vi "Get Annotation Style.vi"(0 "TTLControl in":refnum<class "TTLController.lvclass">, 11 "error in (no error)":errorcluster) -> (4 "TTLControl out":refnum<class "TTLController.lvclass">, 6 "Name":string, 8 "Style":T1, 10 "Active":bool, 15 "error out":errorcluster)   [LabVIEW 2015, in "TTLController.lvclass"]
uses:
  TTLController.lvclass
  FSM Graph VIs/LV Source/Classes/FSM.Annotation/Annotation Style.ctl
  TTLController.lvclass/TTLController.ctl
  FSM Graph VIs/LV Source/Classes/FSM.Annotation/FSM.Annotation.lvclass
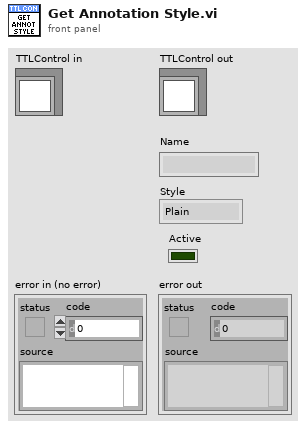
[diagram p1: front panel]
types:
  T1 = typedef "FSM.Annotation.lvclass/Annotation Style.ctl" = enum16{"Plain", "On", "Off", "On-Off"}
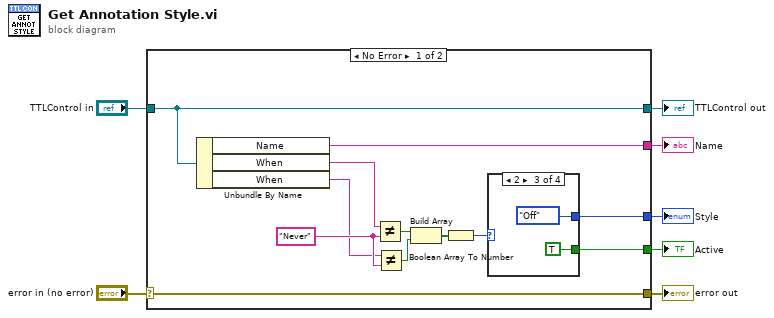
[diagram p0: block diagram]
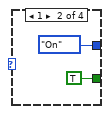
[diagram p3: hidden frame]
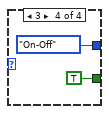
[diagram p4: hidden frame]
diagram:
  n1 = case shown="No Error" "error in (no error)" {
    selector: "error in (no error)" -> [w19 w27]
    tunnel: [w19 w27] -> w6
    tunnel: [w18 w26] -> w4
    tunnel: "TTLControl in" -> [w18 w26]
    tunnel: [w17 _] -> w3
    tunnel: [w9 _] -> w2
    tunnel: [w8 _] -> w1
    frame No Error {
      w13 = "Never" ("y")
      n2 = Unbundle By Name(w18) -> ("Name"=w17:string, "When"=w12:string, "When"=w11:string)
      n3 = Not Equal?(x=w12, y=w13) -> (x != y?=w14:bool)
      n4 = Not Equal?(x=w11, y=w13) -> (x != y?=w16:bool)
      n5 = Build Array(w14, w16) -> (w15:bool[])
      n6 = Boolean Array To Number(Boolean array=w15) -> (number=w10:u32)
      n7 = case shown="2" w10 {
        tunnel: [_ TRUE TRUE TRUE] -> w9
        tunnel: [_ Annotation_Style."On" ("Style") Annotation_Style."Off" ("Style") Annotation_Style."On-Off" ("Style")] -> w8
        frame 0, Default {
        }
        frame 1 {
        }
        frame 2 {
        }
        frame 3 {
        }
      }
    }
    frame Error {
    }
  }
  "error out" <- w6
  "TTLControl out" <- w4
  "Style" <- w1
  "Active" <- w2
  "Name" <- w3
